vi "Write Step Iterations.vi"(8 "error in (no error)":errorcluster, 10 "Step Iterations":refnum<vi>, 11 "Measurement UI in":refnum<class "Measurement UI.lvclass">) -> (0 "error out":errorcluster, 3 "Measurement UI out":refnum<class "Measurement UI.lvclass">)   [LabVIEW 2017, in "Measurement UI.lvlib" / "Measurement UI.lvclass"]
uses:
  Measurement UI.lvclass
  Measurement UI.lvclass/Measurement UI.ctl
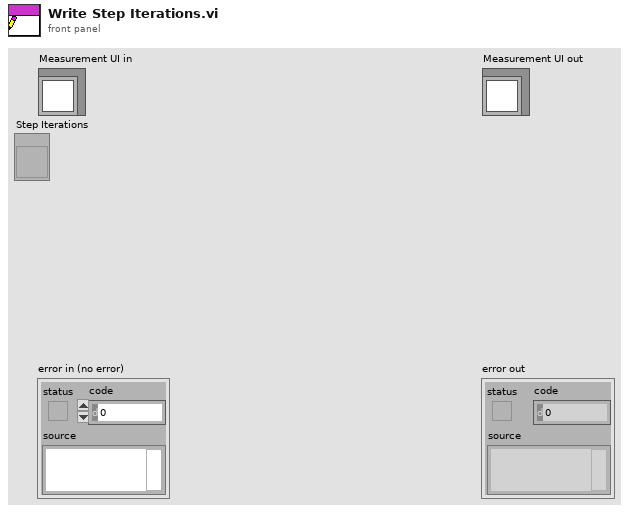
[diagram p1: front panel]
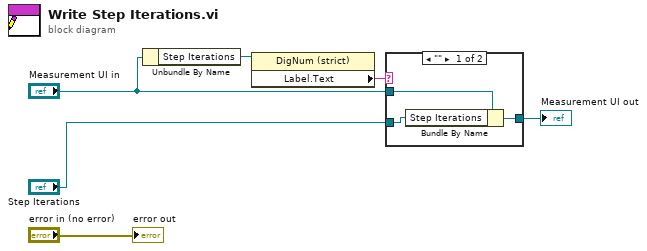
[diagram p0: block diagram]
diagram:
  n1 = Unbundle By Name("Measurement UI in") -> ("Step Iterations"=w6:refnum<vi>)
  n2 = property class="DigNum (strict)"(reference=w6) -> ("Label.Text"=w5:string)  [unwired: 1 in, 2 out]
  n3 = case shown="\"\"" w5 {
    tunnel: [w8 w10] -> w3
    tunnel: "Measurement UI in" -> [w9 w10]
    tunnel: "Step Iterations" -> [w7 _]
    frame "" {
      n4 = Bundle By Name(cluster=w9, "Step Iterations"=w7) -> (w8:refnum<class "Measurement UI.lvclass">)
    }
    frame Default {
    }
  }
  "Measurement UI out" <- w3
  "error out" <- "error in (no error)"
